vi "Add Cosntraint.vi"(8 "error in (no error)":errorcluster, 10 "Check":refnum<class "Constraint.lvclass">, 11 "Check Manager in":refnum<class "Constraint Manager.lvclass">) -> (0 "error out":errorcluster, 3 "Check Manager out":refnum<class "Constraint Manager.lvclass">)   [LabVIEW 2020, in "Composed Columns.lvlib" / "Constraint Manager.lvclass"]
uses:
  Constraint Manager.lvclass
  Check/Constraint.lvclass
  Constraint Manager.lvclass/Constraint Manager.ctl
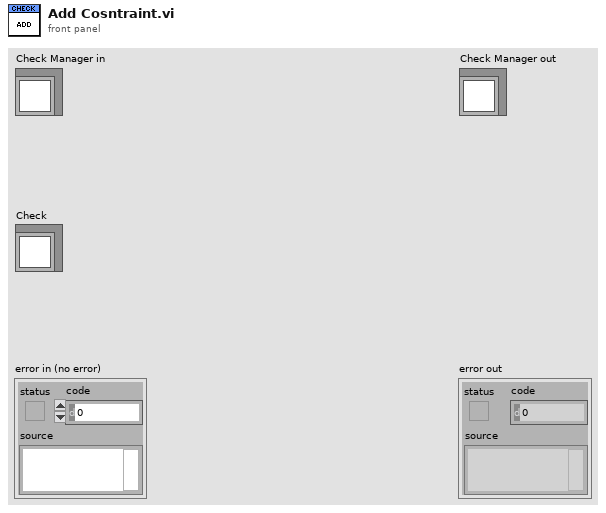
[diagram p1: front panel]
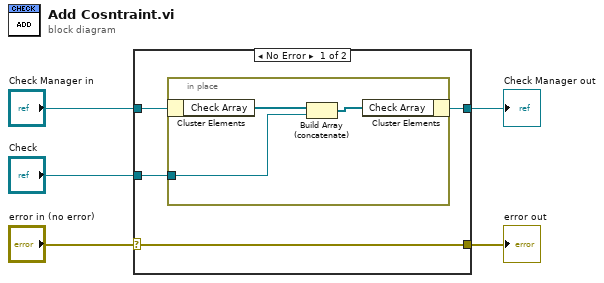
[diagram p0: block diagram]
diagram:
  n1 = case shown="No Error" "error in (no error)" {
    selector: "error in (no error)" -> [w9 w14]
    tunnel: [w9 w14] -> w4
    tunnel: [w7 w13] -> w2
    tunnel: "Check Manager in" -> [w8 w13]
    tunnel: "Check" -> [w6 _]
    frame No Error {
      n2 = in-place {
        in-place-border: w6 -> [w11]
        n3 = in-place-cluster #1(w8) -> ("Check Array"=w12:refnum<class "Constraint.lvclass">[])
        n4 = Build Array (concatenate)(w12, w11) -> (w10:refnum<class "Constraint.lvclass">[])
        n5 = in-place-cluster #1("Check Array"=w10) -> (w7:refnum<class "Constraint Manager.lvclass">)
      }
    }
    frame Error {
    }
  }
  "error out" <- w4
  "Check Manager out" <- w2
